vi "writeSGL.vi"(8 "error in (no error)":errorcluster, 10 "Input":sgl, 11 "ModbusBuffer in":refnum<class "ModbusBuffer.lvclass">) -> (0 "error out":errorcluster, 3 "ModbusBuffer out":refnum<class "ModbusBuffer.lvclass">)   [LabVIEW 2016, in "RTModbus.lvlib" / "ModbusBuffer.lvclass"]
uses:
  ModbusBuffer.lvclass
  ModbusBuffer.lvclass/ModbusBuffer.ctl
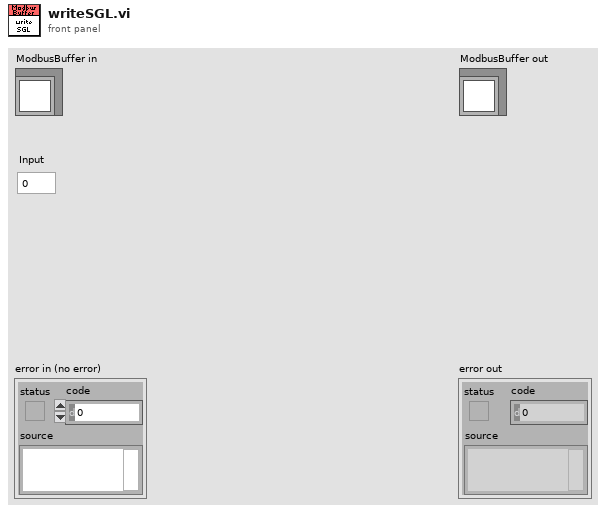
[diagram p1: front panel]
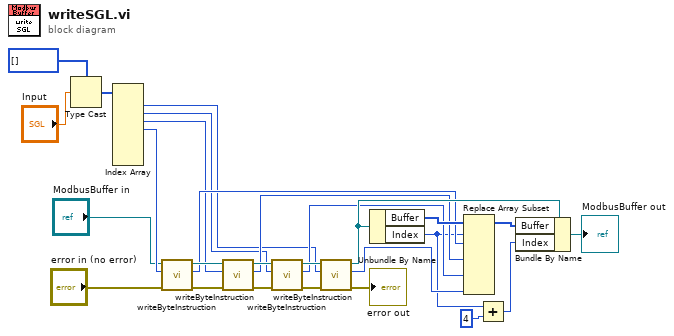
[diagram p0: block diagram]
diagram:
  n1 = Type Cast(type=u8[] [], x="Input") -> (*(type *) &x=w8:u8[])
  n2 = Index Array(array=w8) -> (element #1=w7:u8, element #2=w6:u8, element #3=w5:u8, element #4=w4:u8)  [unwired: 8 in, 4 out]
  n3 = call "writeByteInstruction.vi"("error in (no error)"="error in (no error)", "Input"=w4, "ModbusBuffer in"="ModbusBuffer in") -> ("error out"=w16:errorcluster, "Output"=w11:u16, "ModbusBuffer out"=w22:refnum<class "ModbusBuffer.lvclass">)  [unwired: 6 in]
  n4 = call "writeByteInstruction.vi"("error in (no error)"=w16, "Input"=w5, "ModbusBuffer in"=w22) -> ("error out"=w15:errorcluster, "Output"=w12:u16, "ModbusBuffer out"=w21:refnum<class "ModbusBuffer.lvclass">)  [unwired: 6 in]
  n5 = call "writeByteInstruction.vi"("error in (no error)"=w15, "Input"=w6, "ModbusBuffer in"=w21) -> ("error out"=w14:errorcluster, "Output"=w18:u16, "ModbusBuffer out"=w20:refnum<class "ModbusBuffer.lvclass">)  [unwired: 6 in]
  n6 = call "writeByteInstruction.vi"("error in (no error)"=w14, "Input"=w7, "ModbusBuffer in"=w20) -> ("error out"=→"error out":errorcluster, "Output"=w17:u16, "ModbusBuffer out"=w19:refnum<class "ModbusBuffer.lvclass">)  [unwired: 6 in]
  n7 = Unbundle By Name(w19) -> ("Buffer"=w25:u16[], "Index"=w1:i32)
  n8 = Replace Array Subset(array=w25, new element #1=w11, index #1=w1, new element #2=w12, new element #3=w18, new element #4=w17) -> (w24:u16[])  [unwired: 3 in]
  n9 = Add(x=w1, y=4) -> (x+y=w26:i32)
  n10 = Bundle By Name(cluster=w19, "Buffer"=w24, "Index"=w26) -> (→"ModbusBuffer out":refnum<class "ModbusBuffer.lvclass">)
